vi "Validate Holding Register Mapping.vi"(8 "error in (no error)":errorcluster, 10 "Mapping":u16) -> (0 "error out":errorcluster, 1 "Status Message":string, 3 "Valid?":bool)   [LabVIEW 2015]
uses:
  Modbus Master System Explorer.lvlib
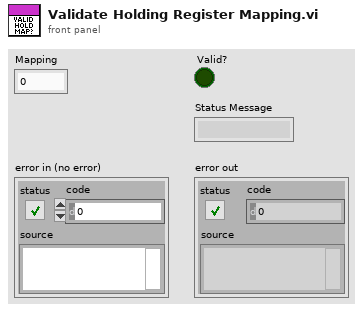
[diagram p1: front panel]
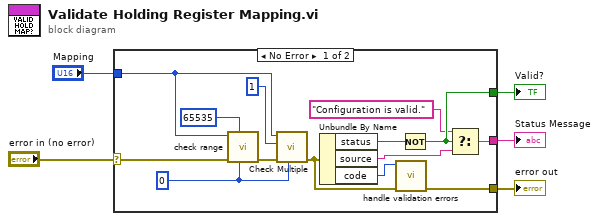
[diagram p0: block diagram]
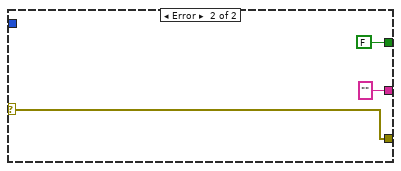
[diagram p2: hidden frame]
diagram:
  n1 = case shown="No Error" "error in (no error)" {
    selector: "error in (no error)" -> [w13 w22]
    tunnel: "Mapping" -> [w9 _]
    tunnel: [w6 w22] -> w3
    tunnel: [w17 FALSE] -> w2
    tunnel: [w14 "" ("source")] -> w1
    frame No Error {
      w10 = 0 ("lower limit")
      n2 = call "check range.vi"("lower limit"=w10, "upper limit"=65535, "error in (no error)"=w13, "Mapping"=w9) -> ("error out"=w12:errorcluster)  [unwired: 7 in]
      n3 = call "Check Multiple.vi"("Offset"=w10, "error in (no error)"=w12, "Divisor"=1 ("y"), "Mapping"=w9) -> ("error out"=w7:errorcluster)  [unwired: 7 in]
      n4 = Unbundle By Name(w7) -> ("status"=w18:bool, "source"=w15:string, "code"=w8:i32)
      n5 = call "handle validation errors.vi"("error in (no error)"=w7, "code"=w8) -> ("error out"=w6:errorcluster)  [unwired: 9 in]
      n6 = Not(x=w18) -> (.not. x?=w17:bool)
      n7 = Select(t="Configuration is valid." ("source"), s=w17, f=w15) -> (s? t:f=w14:string)
    }
    frame Error {
    }
  }
  "error out" <- w3
  "Valid?" <- w2
  "Status Message" <- w1
